vi "lab5_midpoint.vi"(0 "a":dbl, 1 "b":dbl, 2 "Array":dbl[][](array[numeric]), 3 "конец по времени":dbl, 4 "шаг по времени":dbl) -> (5 "Array out":dbl[](array[numeric]))   [LabVIEW 2018]
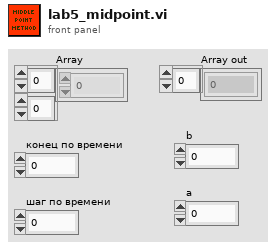
[diagram p1: front panel]
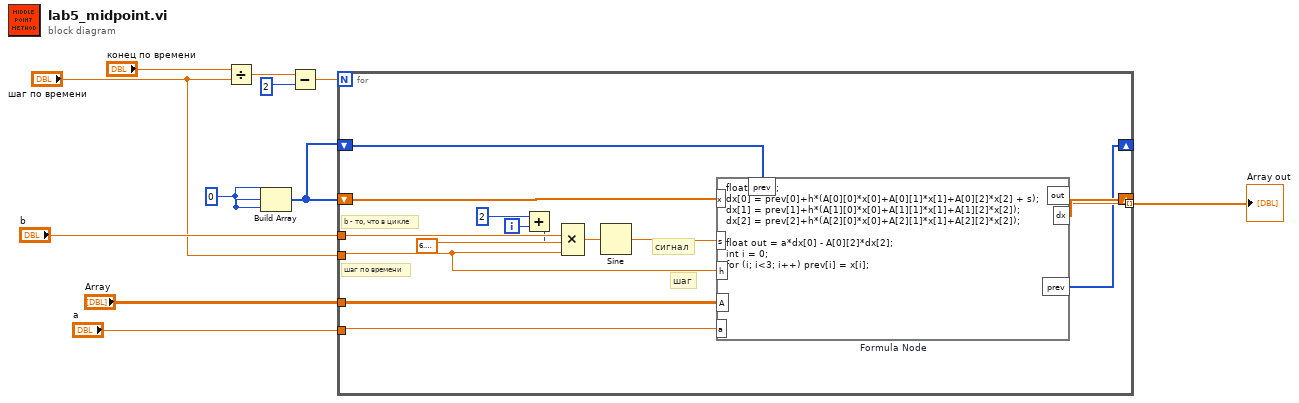
[diagram p0: block diagram]
diagram:
  w6 = 0
  n1 = Divide(x="конец по времени", y="шаг по времени") -> (x/y=w3:dbl)
  n2 = Build Array(w6, w6, w6) -> (w1:i32[])
  n3 = Subtract(x=w3, y=2) -> (x-y=w2:dbl)
  n4 = for {
    N: w2 -> [_]
    tunnel: "b" -> [w25]
    tunnel: "шаг по времени" -> [w22]
    tunnel: [w21] -> w9 mode=indexing
    shift-right: [w23] -> _
    shift-left: w1 -> [w24]
    tunnel: "a" -> [w19]
    tunnel: "Array" -> [w18]
    shift-right: [w12] -> _
    shift-left: w1 -> [w13]
    i -> [w15]
    # "шаг по времени"
    # "b - то, что в цикле"
    # "шаг"
    # "сигнал"
    n5 = Add(x=2, y=w15) -> (x+y=w14:i32)
    n6 = Compound Arithmetic op=MULTIPLY(6.283185307179586, w25, w14, w22) -> (w17:dbl)
    n7 = Sine(x=w17) -> (sin(x)=w20:dbl)
    n8 = formula code="float dx[3];\ndx[0] = prev[0]+h*(A[0][0]*x[0]+A[0][1]*x[1]+A[0][2]*x[2] + s);\ndx[1] = prev[1]+h*(A[1][0]*x[0]+A[1][1]*x[1]+A[1][2]*x[2]);\ndx[2] = prev[2]+h*(A[2][0]*x[0]+A[2][1]*x[1]+A[2][2]*x[2]);\n\nfloat out = a*dx[0] - A[0][2]*dx[2];\nint i = 0;\nfor (i; i<3; i++) prev[i] = x[i];"("x"=w24, "s"=w20, "h"=w22, "A"=w18, "a"=w19, "prev"=w13) -> ("dx"=w23:dbl[], "out"=w21:dbl, "prev"=w12:i32[])
  }
  "Array out" <- w9
